vi "Align Status Buffers.vi"(8 "error in (no error)":errorcluster, 10 "Data Ref":T1, 11 "VeriStand DSF in":refnum<class "VeriStand DSF.lvclass">) -> (0 "error out":errorcluster, 3 "VeriStand DSF out":refnum<class "VeriStand DSF.lvclass">)   [LabVIEW 2020, in "DSF Engine.lvlib" / "VeriStand DSF.lvclass"]
uses:
  VeriStand DSF.lvclass
  <vilib>/NI VeriStand/Custom Device API/Data Table Ref.ctl
  VeriStand DSF.lvclass/VeriStand DSF.ctl
  Includes/DSF Core.lvlibp/Classes/Buffer/Buffer.lvclass
  <vilib>/NI VeriStand/Custom Device API/Custom Device API.lvlib
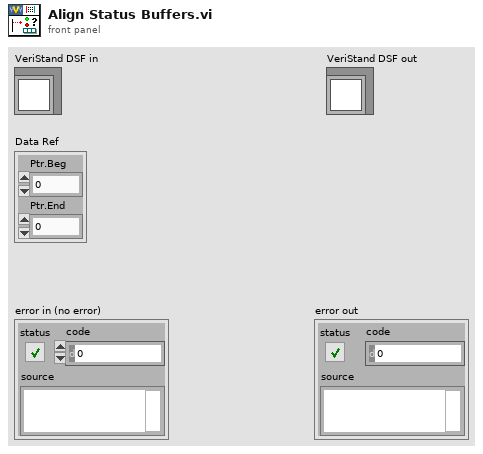
[diagram p1: front panel]
types:
  T1 = typedef "Custom Device API.lvlib/Data Table Ref.ctl" = cluster{"Ptr.Beg":u64, "Ptr.End":u64}
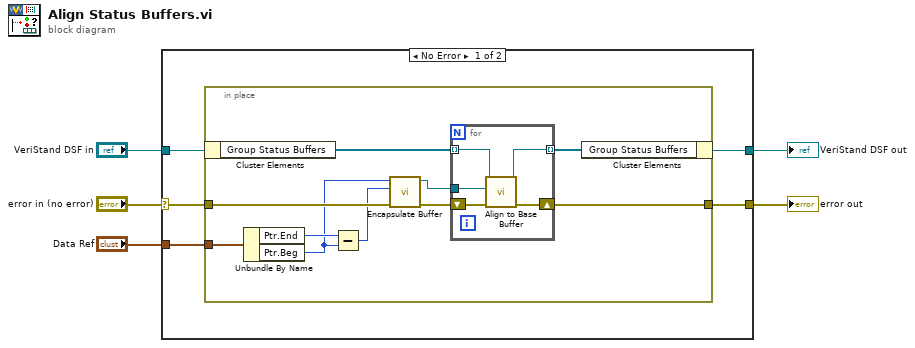
[diagram p0: block diagram]
diagram:
  n1 = case shown="No Error" "error in (no error)" {
    selector: "error in (no error)" -> [w8 w27]
    tunnel: [w7 w27] -> w4
    tunnel: "VeriStand DSF in" -> [w10 w26]
    tunnel: [w9 w26] -> w2
    tunnel: "Data Ref" -> [w6 _]
    frame No Error {
      n2 = in-place {
        in-place-border: w8 -> [w15]
        in-place-border: [w18] -> w7
        in-place-border: w6 -> [w17]
        n3 = in-place-cluster #1(w10) -> ("Group Status Buffers"=w20:refnum<class "Buffer.lvclass">[])
        n4 = Unbundle By Name(w17) -> ("Ptr.End"=w16:u64, "Ptr.Beg"=w12:u64)
        n5 = Subtract(x=w16, y=w12) -> (x-y=w13:u64)
        n6 = call "Encapsulate Buffer.vi"("error in (no error)"=w15, "buffer size"=w13, "buffer address"=w12) -> ("error out"=w14:errorcluster, "Buffer"=w11:refnum<class "Buffer.lvclass">)  [unwired: 7 in]
        n7 = for {
          tunnel: w20 -> [w25] mode=indexing
          tunnel: [w24] -> w19 mode=indexing
          tunnel: w11 -> [w21]
          shift-right: [w23] -> w18
          shift-left: w14 -> [w22]
          n8 = call "Align to Base Buffer.vi"("error in (no error)"=w22, "base Buffer"=w21, "Buffer in"=w25) -> ("error out"=w23:errorcluster, "Buffer out"=w24:refnum<class "Buffer.lvclass">)  [unwired: 7 in]
        }
        n9 = in-place-cluster #1("Group Status Buffers"=w19) -> (w9:refnum<class "VeriStand DSF.lvclass">)
      }
    }
    frame Error {
    }
  }
  "error out" <- w4
  "VeriStand DSF out" <- w2
